vi "Untitled 2.vi"() -> (0 "Tensão Fase B":dynamicdata(graph), 1 "Corrente Fase B":dynamicdata(graph), 2 "Correnmte Fase A":dynamicdata(graph), 4 "Waveform Graph":dynamicdata(graph), 5 "Corrente Fase C":dynamicdata(graph), 6 "Tensão Fase C":dynamicdata(graph))   [LabVIEW 2024]
panel:
  out "Tensão fase A":dynamicdata(graph)
  out "Fase C":string[][](table)
  out "Fase B":string[][](table)
  out "Fase A":string[][](table)
  out "Timestamp":string[][](table)
  out "Waveform Graph 2":dynamicdata(graph)
  out "All data":string[][](table)
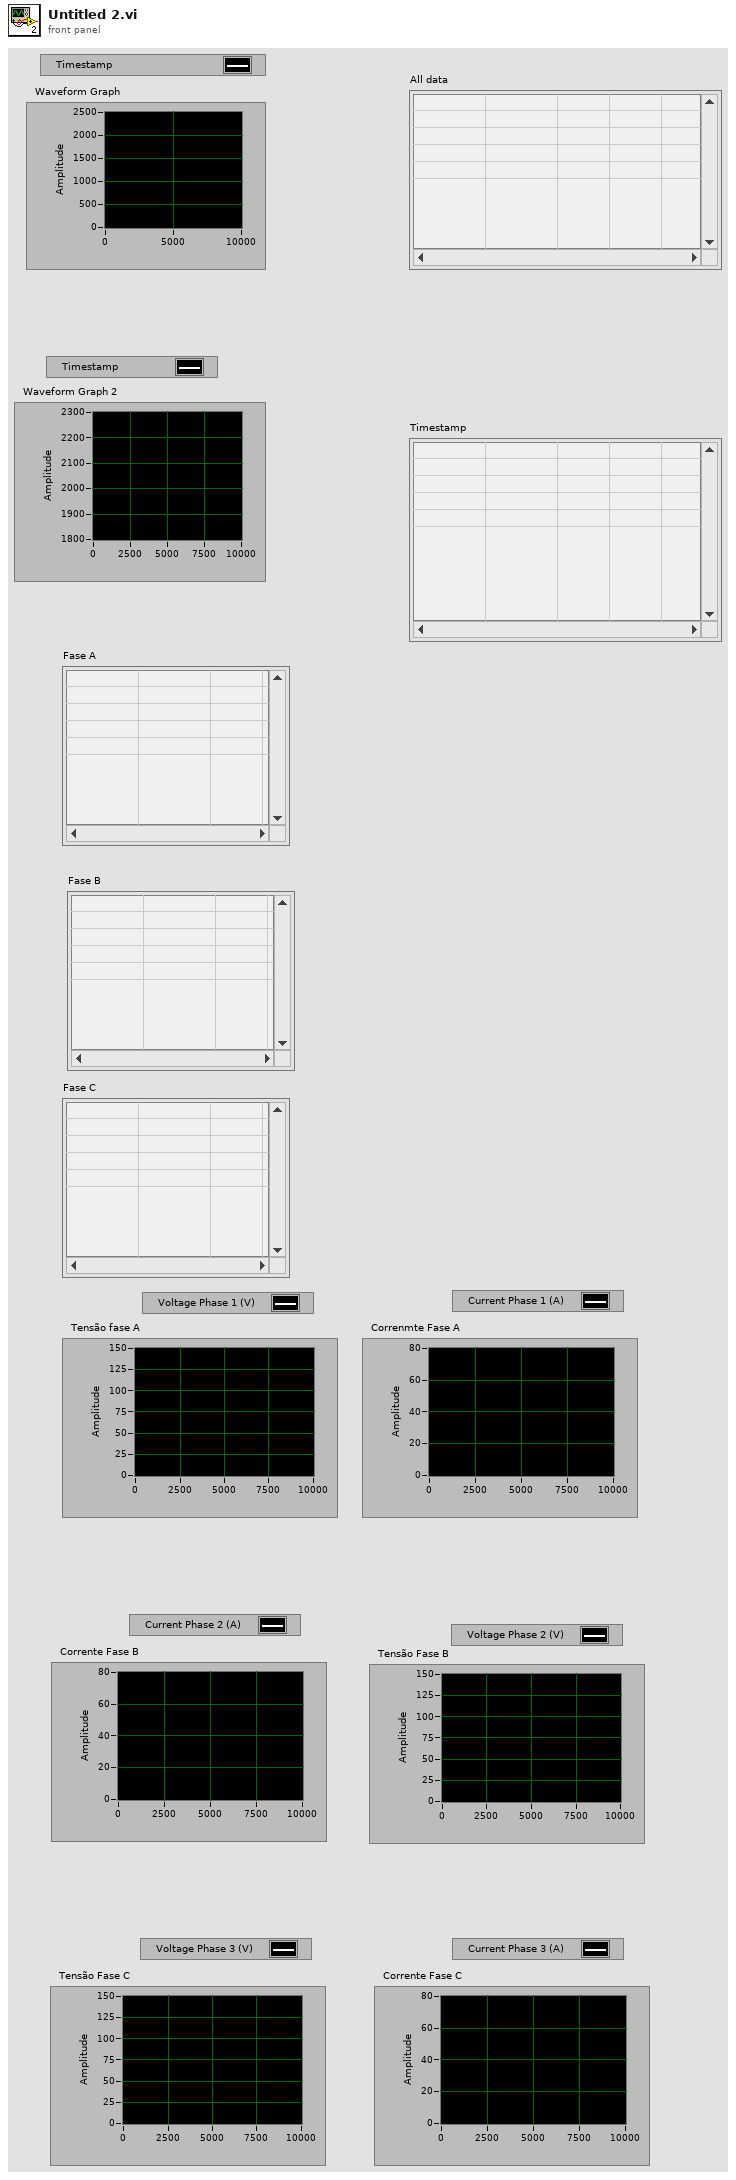
[diagram p1: front panel]
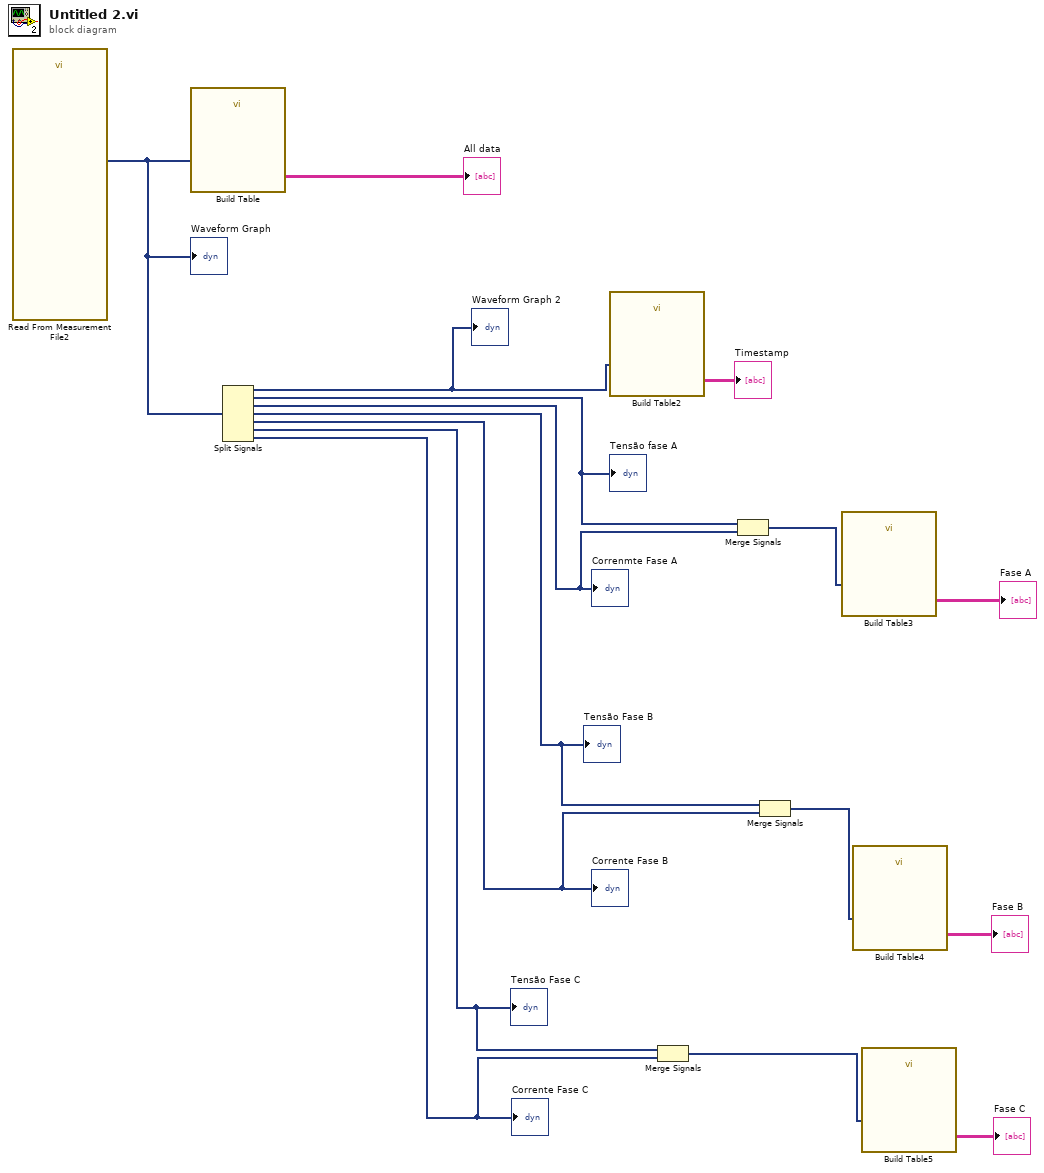
[diagram p0: block diagram]
diagram:
  n1 = call "Read From Measurement File2"() -> ("Signals"=w15:dynamicdata)  [unwired: 6 in, 5 out]
  "Waveform Graph" <- w15
  n2 = call "Build Table"("Signals"=w15) -> ("Table"=→"All data":string[][])  [unwired: 4 in, 6 out]
  n3 = Split Signals(w15) -> (w13:dynamicdata, w12:dynamicdata, w11:dynamicdata, w5:dynamicdata, w4:dynamicdata, w2:dynamicdata, w1:dynamicdata)  [unwired: 7 in]
  "Waveform Graph 2" <- w13
  "Correnmte Fase A" <- w11
  "Corrente Fase B" <- w4
  "Corrente Fase C" <- w1
  "Tensão fase A" <- w12
  "Tensão Fase B" <- w5
  "Tensão Fase C" <- w2
  n4 = call "Build Table2"("Signals"=w13) -> ("Table"=→"Timestamp":string[][])  [unwired: 4 in, 6 out]
  n5 = Merge Signals(w2, w1) -> (w7:dynamicdata)
  n6 = Merge Signals(w12, w11) -> (w10:dynamicdata)
  n7 = Merge Signals(w5, w4) -> (w8:dynamicdata)
  n8 = call "Build Table3"("Signals"=w10) -> ("Table"=→"Fase A":string[][])  [unwired: 4 in, 6 out]
  n9 = call "Build Table4"("Signals"=w8) -> ("Table"=→"Fase B":string[][])  [unwired: 4 in, 6 out]
  n10 = call "Build Table5"("Signals"=w7) -> ("Table"=→"Fase C":string[][])  [unwired: 4 in, 6 out]
